vi "setVss.vi"(11 "index":i32) -> ()   [LabVIEW 2016]
uses:
  variables/imageSettings.vi
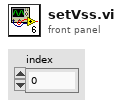
[diagram p1: front panel]
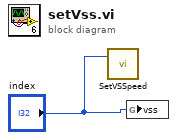
[diagram p0: block diagram]
diagram:
  n1 = call <userlib>:"SetVSSpeed.vi"("index"="index") -> ()  [unwired: 1 in, 2 out]
  n2 = global write "imageSettings.vi" "vss"("index") -> ()
